vi "INIaddStringHash.vi"() -> ()   [LabVIEW 2022 SP3]
uses:
  <vilib>/Utility/config.llb/Write Key (String).vi
  <vilib>/Utility/config.llb/NI_LVConfig.lvlib
panel:
  in  "Error In":errorcluster
  out "Error Out":errorcluster
  in  "SectionName":string
  in  "File Path Control":path
  in  "String":string
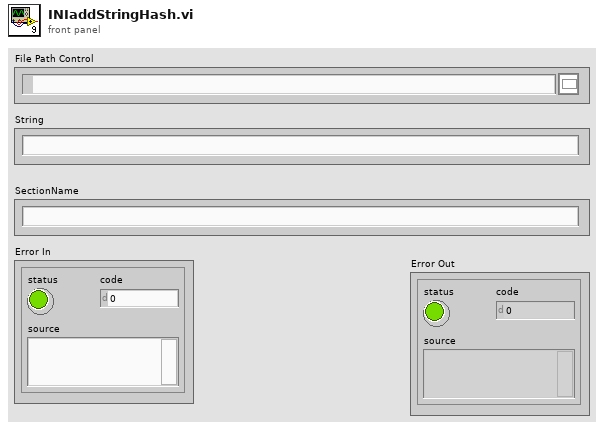
[diagram p1: front panel]
types:
  T1 = typedef "NI_LVConfig.lvlib/Config Data RefNum.ctl" = refnum<k1>
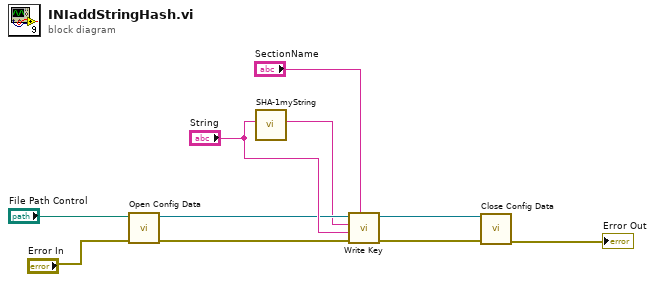
[diagram p0: block diagram]
diagram:
  n1 = call <vilib>:"Open Config Data.vi"("error in (no error)"="Error In", "configuration file path"="File Path Control") -> ("error out"=w6:errorcluster, "refnum"=w8:T1)  [unwired: 7 in, 1 out]
  n2 = call "SHA-1myString.vi"("HashThis"="String") -> ("SHA1string"=w3:string)  [unwired: 9 in, 1 out]
  n3 = call-poly <vilib>:"Write Key.vi"("section"="SectionName", "error in (no error)"=w6, "value"="String", "key"=w3, "refnum"=w8) -> ("error out"=w5:errorcluster, "refnum out"=w4:T1)  [unwired: 4 in, 1 out]
  n4 = call <vilib>:"Close Config Data.vi"("error in (no error)"=w5, "refnum"=w4) -> ("error out"=→"Error Out":errorcluster)  [unwired: 8 in, 1 out]
